vi "_Last Ack Event.vi"(10 "Event":refnum<class "Event.lvclass">) -> (3 "Last Ack Event Msg Strategy out":refnum<class "Last Ack Event Msg Strategy.lvclass">)   [LabVIEW 2021, in "jettl.lvlib" / "jettl Msg Last Ack Event.lvlib"]
uses:
  jettl Msg Last Ack Event.lvlib
  Event/Event.lvclass
  Last Ack Event Msg Strategy/Last Ack Event Msg Strategy.lvclass
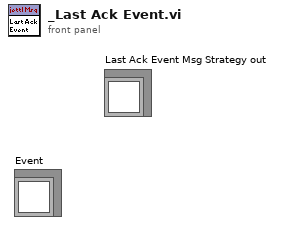
[diagram p1: front panel]
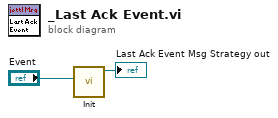
[diagram p0: block diagram]
diagram:
  n1 = call "Init.vi"("Event"="Event") -> ("Last Ack Event Msg Strategy out"=→"Last Ack Event Msg Strategy out":refnum<class "Last Ack Event Msg Strategy.lvclass">)  [unwired: 10 in]
